vi "Channel Performance Test.vi"() -> ()   [LabVIEW 2021]
uses:
  Double/CIF_NIChn_Double.lvclass
  <vilib>/Platform/TimedLoop/XDataNode/timing_clust.ctl
  <vilib>/Platform/TimedLoop/XDataNode/nitl_modes.ctl
  <vilib>/Platform/TimedLoop/XDataNode/wakeup.ctl
  CIFChannels/Typedef/Direction.ctl
  7d13c5b7-0b44-4ab4-8a6c-0bcd63b70b59.vi
  c0ba1b46-a5a0-42bd-afb3-2f6832d2a88c.vi
  6a1b8880-d4c2-444f-a4b2-811244e6db06.vi
  10e1b524-69ef-478e-ae98-36060d5eb0d6.vi
  332321e3-b478-4438-b8ac-43cf378b23bb.vi
  <vilib>/CIFChannels/SubVIs/Add Error.vi
  7d13c5b7-0b44-4ab4-8a6c-0bcd63b70b59.vi/c28b0ead-42ad-4072-80a2-aca7f2bd7ce3.vi
  <vilib>/CIFChannels/SubVIs/CIFServices Fill In Error Info Ex.vi
  <vilib>/CIFChannels/SubVIs/Get dll Path.vi
  c0ba1b46-a5a0-42bd-afb3-2f6832d2a88c.vi/4bc1c15b-36ab-481f-b8dd-c64075ce723a.vi
  c0ba1b46-a5a0-42bd-afb3-2f6832d2a88c.vi/d83cb72b-7713-41fc-a3d1-682de79cf574.vi
  6a1b8880-d4c2-444f-a4b2-811244e6db06.vi/c28b0ead-42ad-4072-80a2-aca7f2bd7ce3.vi
  10e1b524-69ef-478e-ae98-36060d5eb0d6.vi/c28b0ead-42ad-4072-80a2-aca7f2bd7ce3.vi
  10e1b524-69ef-478e-ae98-36060d5eb0d6.vi/219d0231-d98b-4193-b5cc-84f90e3c9091.vi
  332321e3-b478-4438-b8ac-43cf378b23bb.vi/c28b0ead-42ad-4072-80a2-aca7f2bd7ce3.vi
  332321e3-b478-4438-b8ac-43cf378b23bb.vi/219d0231-d98b-4193-b5cc-84f90e3c9091.vi
  <vilib>/CIFChannels/SubVIs/Append Error Location.vi
  <vilib>/Platform/TimedLoop/XDataNode/XDataNode.xnode
  <vilib>/Platform/TimedLoop/XDataNode/XDNodeRunTimeDep.lvlib
  <vilib>/CIFChannels/CIFChannelCore.lvlib
  CIFChannels/CIFChannels.lvclass
panel:
  out "avg dbl channel":dbl
  out "max dbl channel":dbl
  out "avg raw channel":dbl
  out "max raw channel":dbl
  out "pass":bool
  out "error out":errorcluster
  # "This test should be run on RT.  It stresses the communications by constantly creating resource contraints with the low priority sender and the high priority loop. On Windows the priority of the loops cannot be set."
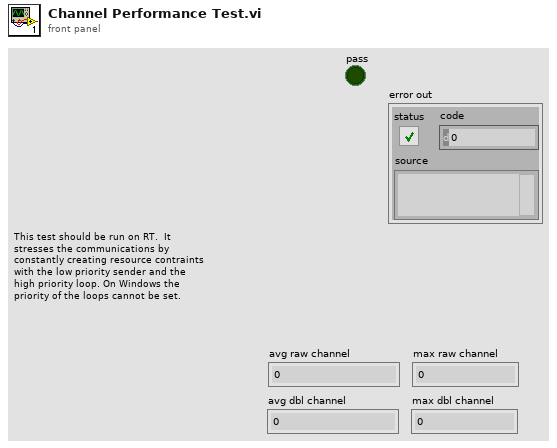
[diagram p1: front panel]
types:
  T1 = typedef "XDNodeRunTimeDep.lvlib/timing_clust.ctl" = cluster{"Expected End [f-1]":u64, "Actual End [f-1]":u64, "Finished Late? [f-1]":bool, "Expected End [i-1]":u64, "Actual End [i-1]":u64, "Finished Late? [i-1]":bool, "Expected Start [i]":u64, "Actual Start [i]":u64, "Expected Start [f]":u64, "Actual Start [f]":u64, "Source Name":string, "Structure Name":string, "Period":i64, "Deadline":i64, "Offset":i64, "Start":i64, "Priority":i32, "Timeout":i32, "Mode":T2, "Wakeup Reason":T3, "Error":errorcluster, "Source Type":string, "Secondary Source Type":string, "Global End Time":u64, "Global Start Time":u64, "Frame Duration":u64, "Iteration Duration":u64, "Assigned CPU":i32, "I/O Scan Engine Mode":u32}
  T2 = typedef "XDNodeRunTimeDep.lvlib/nitl_modes.ctl" = enum32{"No Change", "Process missed periods, maintain original phase", "Discard missed periods, maintain original phase", "Process missed periods, ignore original phase", "Discard missed periods, ignore original phase"}
  T3 = typedef "XDNodeRunTimeDep.lvlib/wakeup.ctl" = enum32{"Normal", "Aborted", "Asynchronous wakeup", "Timing source error", "Timed loop error", "Timeout"}
  T4 = typedef "CIFChannels.lvclass/Direction.ctl" = enum16{"Publisher", "Subscriber"}
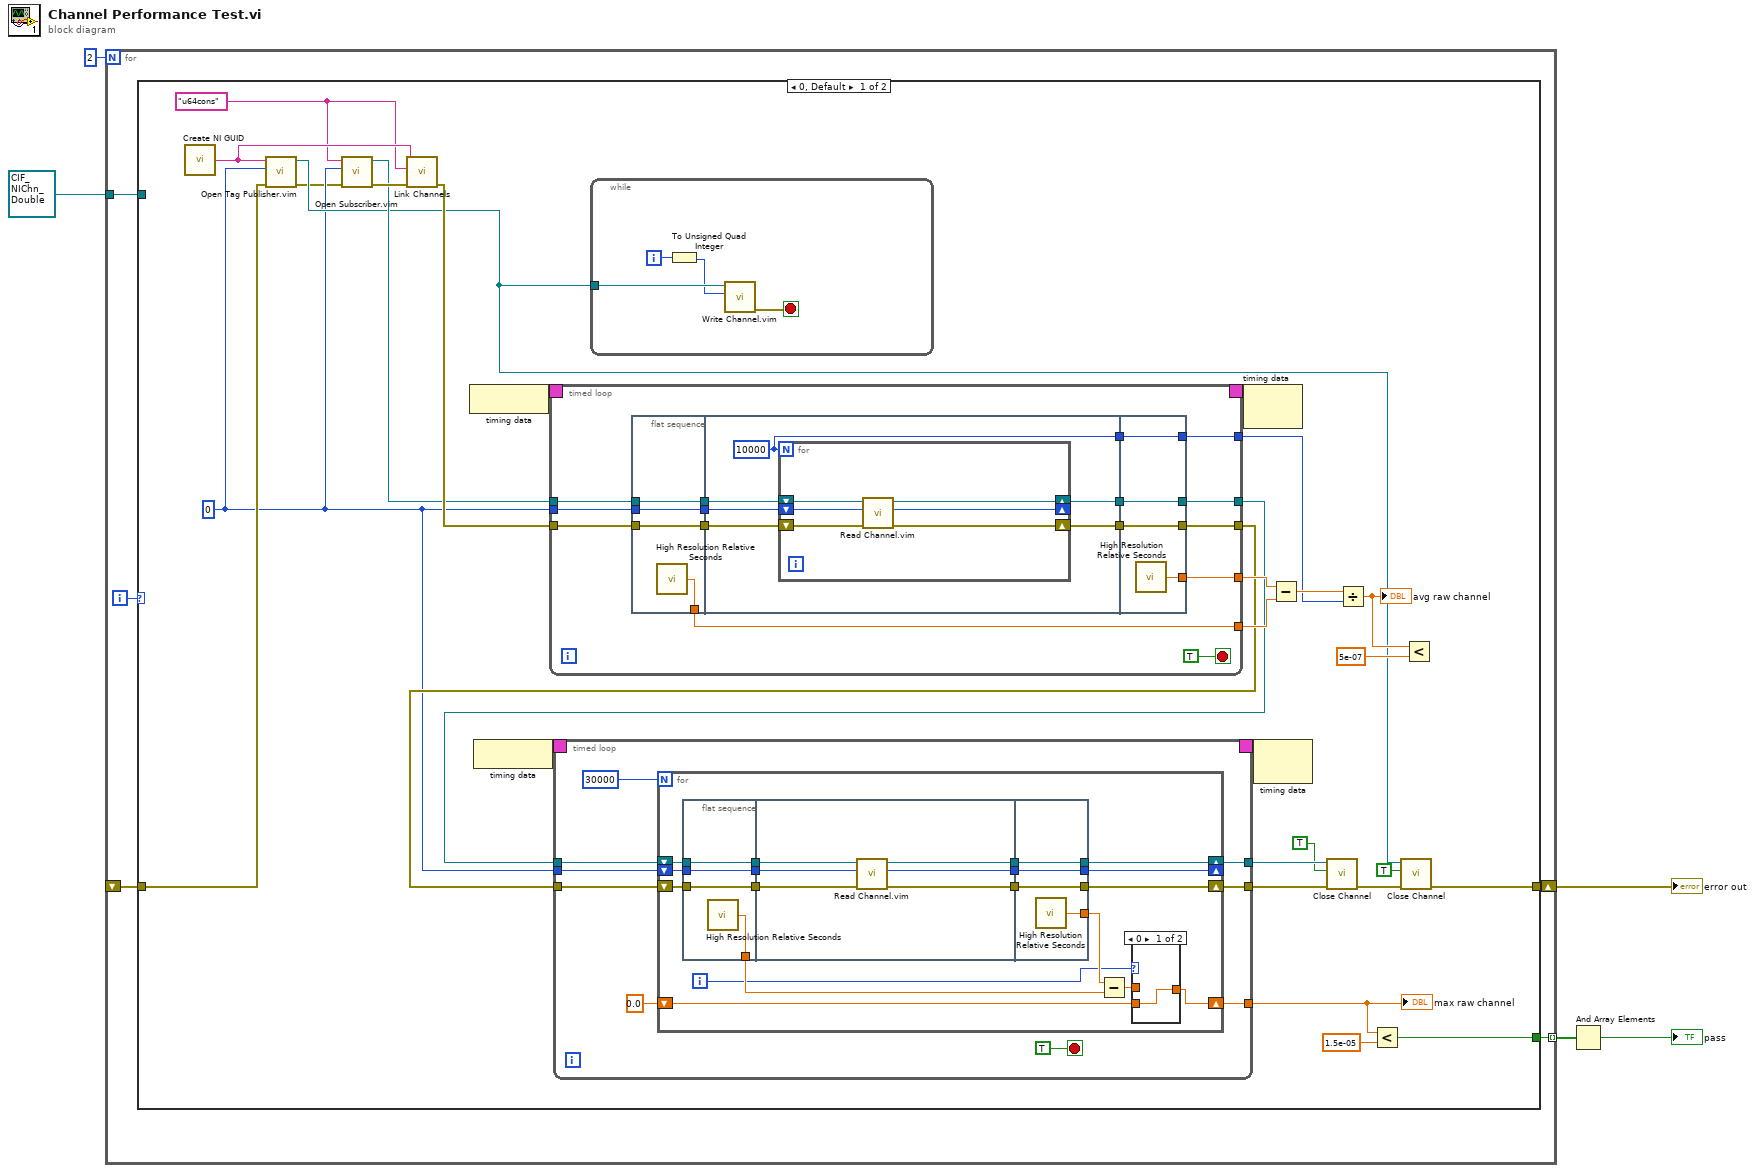
[diagram p0: block diagram]
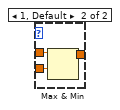
[diagram p2: hidden frame]
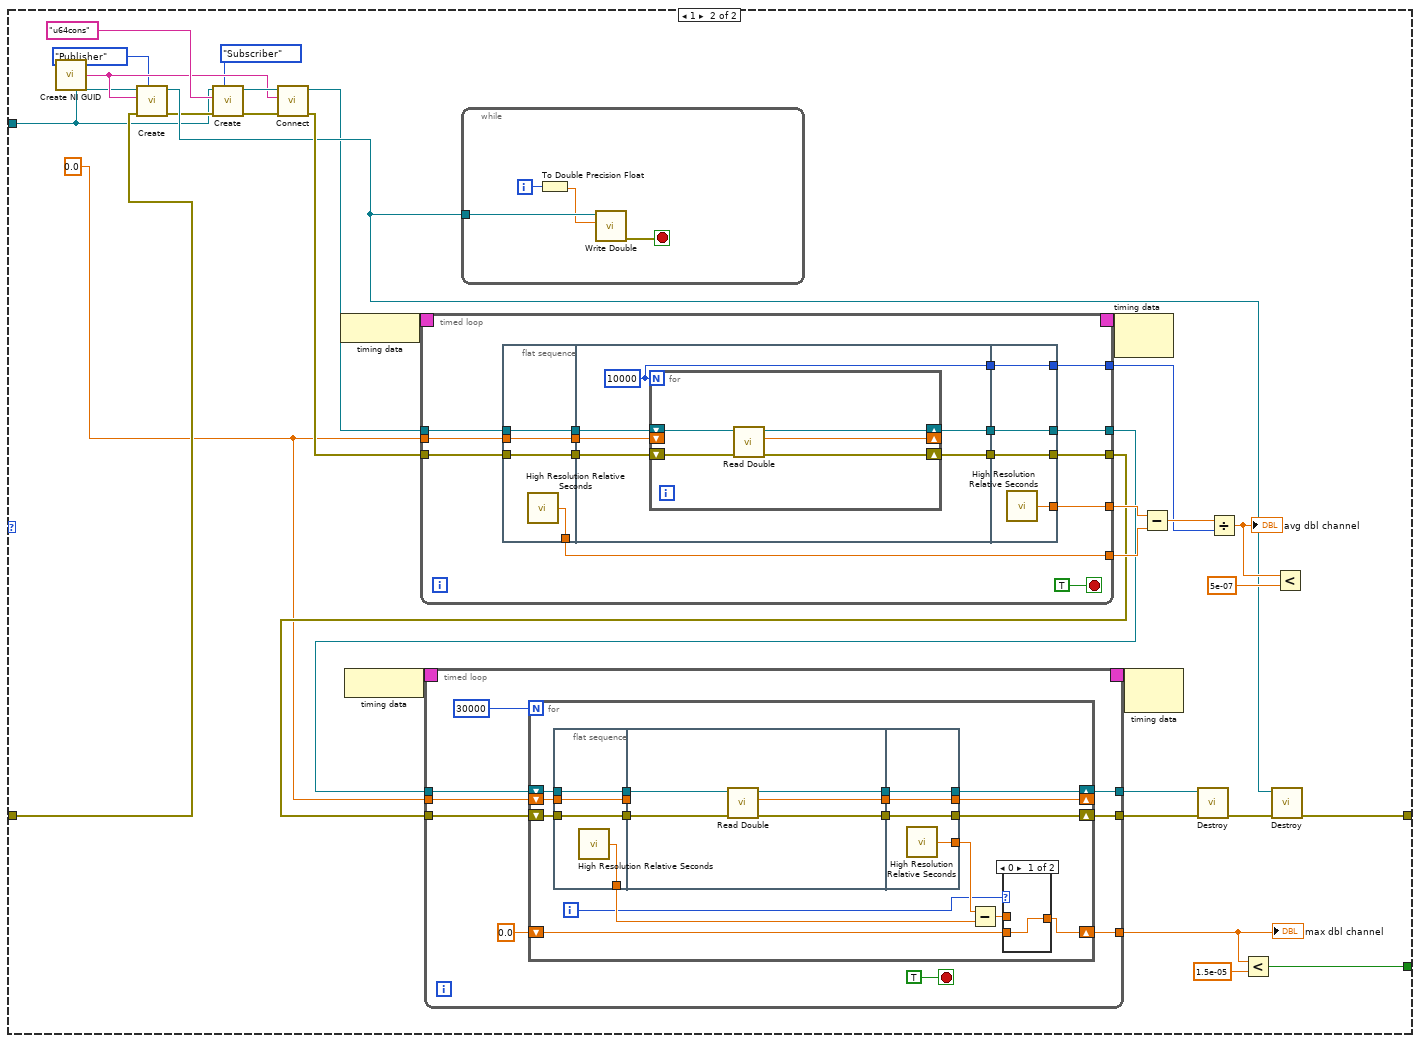
[diagram p3: hidden frame]
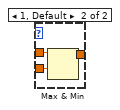
[diagram p4: hidden frame]
diagram:
  n1 = for {
    N: 2 -> [_]
    tunnel: [w10] -> w3 mode=indexing
    shift-right: [w9] -> w5
    shift-left: _ -> [w7]
    tunnel: refnum<class "CIF_NIChn_Double.lvclass"> refnum ("CIF_NIChn_Double.lvclass") -> [w6]
    i -> [w8]
    n2 = case shown="0, Default" w8 {
      tunnel: [w26 w150] -> w10
      tunnel: [w19 w144] -> w9
      tunnel: w7 -> [w24 w148]
      tunnel: w6 -> [_ w134]
      frame 0, Default {
        w14 = "u64cons" ("Channel Name")
        w12 = u64 0
        n3 = call <vilib>:"Create NI GUID.vi"() -> ("NI GUID"=w15:string)
        n4 = call "Open Tag Publisher.vim"("error in"=w24, "Input Type"=w12, "Channel Name"=w15) -> ("error out"=w11:errorcluster, "CIF Channel"=w13:refnum<k21>)  [unwired: 7 in]
        n5 = call "Open Subscriber.vim"("error in"=w11, "Input Type"=w12, "Channel Name"=w14) -> ("error out"=w17:errorcluster, "CIF Channel"=w16:refnum<k21>)  [unwired: 7 in]
        n6 = call <vilib>:"Link Channels.vi"("error in"=w17, "Consumer Channel Name"=w14, "Producer Channel Name"=w15) -> ("error out"=w25:errorcluster)  [unwired: 8 in]
        n7 = node-c288() -> (w40:T1)
        n8 = node-c288() -> (w38:T1)
        n9 = timed-loop {
          timing: w40 -> [_]
          timing-out: [_] -> w39
          tunnel: w16 -> [w108]
          tunnel: w25 -> [w107]
          tunnel: [w103] -> w32
          tunnel: [w101] -> w31
          tunnel: [w99] -> w36
          tunnel: [w98] -> w35
          tunnel: [w97] -> w33
          tunnel: w12 -> [w95]
          stop <- TRUE stop-if-true
          n10 = flat-sequence {
            tunnel: w107 -> [w111]
            tunnel: w108 -> [w112]
            tunnel: [w112] -> w105
            tunnel: [w111] -> w104
            tunnel: [w110] -> w98
            tunnel: w95 -> [w109]
            tunnel: [w109] -> w94
            tunnel: w105 -> [w118]
            tunnel: w104 -> [w117]
            tunnel: [w116] -> w102
            tunnel: [w115] -> w100
            tunnel: [w114] -> w96
            tunnel: w94 -> [w113]
            tunnel: [w128] -> w103
            tunnel: w102 -> [w128]
            tunnel: [w127] -> w101
            tunnel: w100 -> [w127]
            tunnel: [w126] -> w99
            tunnel: [w125] -> w97
            tunnel: w96 -> [w125]
            frame #0 {
              n11 = call <vilib>:"High Resolution Relative Seconds.vi"() -> ("relative seconds"=w110:dbl)
            }
            frame #1 {
              w114 = 10000
              n12 = for {
                N: w114 -> [_]
                shift-right: [w121] -> w116
                shift-left: w118 -> [w124]
                shift-right: [w120] -> w115
                shift-left: w117 -> [w119]
                shift-right: [w122] -> _
                shift-left: w113 -> [w123]
                n13 = call "Read Channel.vim"("error in"=w119, "Data in"=w123, "CIF Channel in"=w124) -> ("error out"=w120:errorcluster, "Data out"=w122:u64, "CIF Channel out"=w121:refnum<k21>)  [unwired: 5 in, 1 out]
              }
            }
            frame #2 {
              n14 = call <vilib>:"High Resolution Relative Seconds.vi"() -> ("relative seconds"=w126:dbl)
            }
          }
        }
        n15 = timed-loop {
          timing: w38 -> [_]
          timing-out: [_] -> w37
          tunnel: w32 -> [w53]
          tunnel: w31 -> [w52]
          tunnel: [w50] -> w22
          tunnel: [w49] -> w23
          tunnel: w12 -> [w48]
          tunnel: [w45] -> w28
          stop <- TRUE stop-if-true
          n16 = for {
            N: 30000 -> [_]
            shift-right: [w65] -> w50
            shift-left: w53 -> [w67]
            shift-right: [w64] -> w49
            shift-left: w52 -> [w66]
            shift-right: [w58] -> w45
            shift-left: 0.0 -> [w59]
            shift-right: [w57] -> _
            shift-left: w48 -> [w63]
            i -> [w55]
            n17 = flat-sequence {
              tunnel: w66 -> [w78]
              tunnel: w67 -> [w79]
              tunnel: [w79] -> w71
              tunnel: [w78] -> w70
              tunnel: [w77] -> w61
              tunnel: w63 -> [w76]
              tunnel: [w76] -> w69
              tunnel: w71 -> [w85]
              tunnel: w70 -> [w81]
              tunnel: [w84] -> w68
              tunnel: w69 -> [w83]
              tunnel: [w82] -> w56
              tunnel: [w80] -> w54
              tunnel: [w89] -> w65
              tunnel: w68 -> [w89]
              tunnel: [w88] -> w64
              tunnel: [w87] -> w62
              tunnel: [w86] -> w57
              tunnel: w56 -> [w86]
              tunnel: w54 -> [w88]
              frame #0 {
                n18 = call <vilib>:"High Resolution Relative Seconds.vi"() -> ("relative seconds"=w77:dbl)
              }
              frame #1 {
                n19 = call "Read Channel.vim"("error in"=w81, "Data in"=w83, "CIF Channel in"=w85) -> ("error out"=w80:errorcluster, "Data out"=w82:u64, "CIF Channel out"=w84:refnum<k21>)  [unwired: 5 in, 1 out]
              }
              frame #2 {
                n20 = call <vilib>:"High Resolution Relative Seconds.vi"() -> ("relative seconds"=w87:dbl)
              }
            }
            n21 = Subtract(x=w62, y=w61) -> (x-y=w60:dbl)
            n22 = case shown="0" w55 {
              tunnel: w60 -> [_ w75]
              tunnel: w59 -> [w72 w74]
              tunnel: [w72 w73] -> w58
              frame 0 {
              }
              frame 1, Default {
                n23 = Max & Min(x=w75, y=w74) -> (max(x,y)=w73:dbl)  [unwired: 1 out]
              }
            }
          }
        }
        "max raw channel" <- w28
        n24 = while {
          tunnel: w13 -> [w43]
          i -> [w44]
          stop <- w41 stop-if-true
          n25 = To Unsigned Quad Integer(1:w44) -> (0:w42:u64)
          n26 = call "Write Channel.vim"("Data in"=w42, "CIF Channel in"=w43) -> ("error out"=w41:errorcluster)  [unwired: 6 in, 3 out]
        }
        n27 = node-c288(w39) -> ()  [unwired: 1 out]
        n28 = node-c288(w37) -> ()  [unwired: 1 out]
        n29 = Subtract(x=w36, y=w35) -> (x-y=w34:dbl)
        n30 = call <vilib>:"Close Channel.vi"("error in"=w23, "Force Destroy? (F)"=TRUE, "CIF Channel"=w22) -> ("error out"=w21:errorcluster)  [unwired: 8 in]
        n31 = Divide(x=w34, y=w33) -> (x/y=w30:dbl)
        "avg raw channel" <- w30
        n32 = Less?(x=w28, y=1.5e-05) -> (x < y?=w26:bool)
        n33 = call <vilib>:"Close Channel.vi"("error in"=w21, "Force Destroy? (F)"=TRUE, "CIF Channel"=w13) -> ("error out"=w19:errorcluster)  [unwired: 8 in]
        n34 = Less?(x=w30, y=5e-07) -> ()  [unwired: 1 out]
      }
      frame 1 {
        w142 = 0.0
        n35 = call <vilib>:"Create NI GUID.vi"() -> ("NI GUID"=w136:string)
        n36 = call-dynamic "Create.vi"("Direction"=Direction."Publisher", "error in (no error)"=w148, "Name"=w136, "CIFTag in"=w134) -> ("error out"=w141:errorcluster, "CIFTag out"=w143:refnum<class "CIF_NIChn_Double.lvclass">)  [unwired: 6 in]
        n37 = call-dynamic "Create.vi"("Direction"=Direction."Subscriber", "error in (no error)"=w141, "Name"="u64cons" ("Channel Name"), "CIFTag in"=w134) -> ("error out"=w139:errorcluster, "CIFTag out"=w138:refnum<class "CIF_NIChn_Double.lvclass">)  [unwired: 6 in]
        n38 = call-dynamic "Connect.vi"("error in (no error)"=w139, "Connection Name"=w136, "CIFTag in"=w138) -> ("error out"=w149:errorcluster, "CIFTag out"=w137:refnum<class "CIF_NIChn_Double.lvclass">)  [unwired: 7 in]
        n39 = node-c288() -> (w164:T1)
        n40 = node-c288() -> (w162:T1)
        n41 = timed-loop {
          timing: w164 -> [_]
          timing-out: [_] -> w163
          tunnel: w137 -> [w231]
          tunnel: w149 -> [w230]
          tunnel: [w226] -> w156
          tunnel: [w224] -> w155
          tunnel: [w222] -> w160
          tunnel: [w221] -> w159
          tunnel: [w220] -> w157
          tunnel: w142 -> [w218]
          stop <- TRUE stop-if-true
          n42 = flat-sequence {
            tunnel: w230 -> [w234]
            tunnel: w231 -> [w235]
            tunnel: [w235] -> w228
            tunnel: [w234] -> w227
            tunnel: [w233] -> w221
            tunnel: w218 -> [w232]
            tunnel: [w232] -> w217
            tunnel: w228 -> [w241]
            tunnel: w227 -> [w240]
            tunnel: [w239] -> w225
            tunnel: [w238] -> w223
            tunnel: [w237] -> w219
            tunnel: w217 -> [w236]
            tunnel: [w250] -> w226
            tunnel: w225 -> [w250]
            tunnel: [w249] -> w224
            tunnel: w223 -> [w249]
            tunnel: [w248] -> w222
            tunnel: [w247] -> w220
            tunnel: w219 -> [w247]
            frame #0 {
              n43 = call <vilib>:"High Resolution Relative Seconds.vi"() -> ("relative seconds"=w233:dbl)
            }
            frame #1 {
              w237 = 10000
              n44 = for {
                N: w237 -> [_]
                shift-right: [w244] -> w239
                shift-left: w241 -> [w246]
                shift-right: [w243] -> w238
                shift-left: w240 -> [w242]
                shift-right: [w245] -> _
                shift-left: w236 -> [_]
                n45 = call-dynamic "Read Double.vi"("error in (no error)"=w242, "CIFTag in"=w246) -> ("error out"=w243:errorcluster, "Data"=w245:dbl, "CIFTag out"=w244:refnum<class "CIF_NIChn_Double.lvclass">)  [unwired: 6 in, 1 out]
              }
            }
            frame #2 {
              n46 = call <vilib>:"High Resolution Relative Seconds.vi"() -> ("relative seconds"=w248:dbl)
            }
          }
        }
        n47 = timed-loop {
          timing: w162 -> [_]
          timing-out: [_] -> w161
          tunnel: w156 -> [w177]
          tunnel: w155 -> [w176]
          tunnel: [w174] -> w146
          tunnel: [w173] -> w147
          tunnel: w142 -> [w172]
          tunnel: [w169] -> w152
          stop <- TRUE stop-if-true
          n48 = for {
            N: 30000 -> [_]
            shift-right: [w189] -> w174
            shift-left: w177 -> [w191]
            shift-right: [w188] -> w173
            shift-left: w176 -> [w190]
            shift-right: [w182] -> w169
            shift-left: 0.0 -> [w183]
            shift-right: [w181] -> _
            shift-left: w172 -> [w187]
            i -> [w179]
            n49 = flat-sequence {
              tunnel: w190 -> [w202]
              tunnel: w191 -> [w203]
              tunnel: [w203] -> w195
              tunnel: [w202] -> w194
              tunnel: [w201] -> w185
              tunnel: w187 -> [w200]
              tunnel: [w200] -> w193
              tunnel: w195 -> [w208]
              tunnel: w194 -> [w205]
              tunnel: [w207] -> w192
              tunnel: w193 -> [_]
              tunnel: [w206] -> w180
              tunnel: [w204] -> w178
              tunnel: [w212] -> w189
              tunnel: w192 -> [w212]
              tunnel: [w211] -> w188
              tunnel: [w210] -> w186
              tunnel: [w209] -> w181
              tunnel: w180 -> [w209]
              tunnel: w178 -> [w211]
              frame #0 {
                n50 = call <vilib>:"High Resolution Relative Seconds.vi"() -> ("relative seconds"=w201:dbl)
              }
              frame #1 {
                n51 = call-dynamic "Read Double.vi"("error in (no error)"=w205, "CIFTag in"=w208) -> ("error out"=w204:errorcluster, "Data"=w206:dbl, "CIFTag out"=w207:refnum<class "CIF_NIChn_Double.lvclass">)  [unwired: 6 in, 1 out]
              }
              frame #2 {
                n52 = call <vilib>:"High Resolution Relative Seconds.vi"() -> ("relative seconds"=w210:dbl)
              }
            }
            n53 = Subtract(x=w186, y=w185) -> (x-y=w184:dbl)
            n54 = case shown="0" w179 {
              tunnel: w184 -> [_ w199]
              tunnel: w183 -> [w196 w198]
              tunnel: [w196 w197] -> w182
              frame 0 {
              }
              frame 1, Default {
                n55 = Max & Min(x=w199, y=w198) -> (max(x,y)=w197:dbl)  [unwired: 1 out]
              }
            }
          }
        }
        "max dbl channel" <- w152
        n56 = while {
          tunnel: w143 -> [w167]
          i -> [w168]
          stop <- w165 stop-if-true
          n57 = To Double Precision Float(number=w168) -> (double precision float=w166:dbl)
          n58 = call-dynamic "Write Double.vi"("Data"=w166, "CIFTag in"=w167) -> ("error out"=w165:errorcluster)  [unwired: 7 in, 2 out]
        }
        n59 = node-c288(w163) -> ()  [unwired: 1 out]
        n60 = node-c288(w161) -> ()  [unwired: 1 out]
        n61 = Subtract(x=w160, y=w159) -> (x-y=w158:dbl)
        n62 = call-dynamic "Destroy.vi"("error in (no error)"=w147, "CIFTag in"=w146) -> ("error out"=w145:errorcluster)  [unwired: 8 in, 1 out]
        n63 = Divide(x=w158, y=w157) -> (x/y=w154:dbl)
        "avg dbl channel" <- w154
        n64 = Less?(x=w152, y=1.5e-05) -> (x < y?=w150:bool)
        n65 = call-dynamic "Destroy.vi"("error in (no error)"=w145, "CIFTag in"=w143) -> ("error out"=w144:errorcluster)  [unwired: 8 in, 1 out]
        n66 = Less?(x=w154, y=5e-07) -> ()  [unwired: 1 out]
      }
    }
  }
  "error out" <- w5
  n67 = And Array Elements(Boolean array=w3) -> (logical AND=→"pass":bool)
